vi "ZAlign_Draw_Locals_DecoFrame.vi"(8 "error in (no error)":errorcluster, 9 "Left":u32, 10 "ControlsAvailable":bool caption="Boolean", 11 "Generic in":refnum<vi>) -> (0 "error out":errorcluster, 3 "Decoration out":refnum<vi>)   [LabVIEW 2014, in "ZAlign.lvlib"]
doc: "ZAlign.lvlib:ZAlign_Draw_Locals_DecoFrame.vi\n----------------------------------------------\nDraw Locals Decoframe\n\nInputs:\n---------------------\n- error in (no error) : Cluster; \n- Left : U32; \n- Boolean : Boolean; \n- Generic in : Refnum; \n\nOutputs:\n---------------------\n- error out : Cluster; \n- Decoration out : Refnum; \n\n----------------------------------------------\n16/03/2015\nZühlke Engineering AG\nCH-8952 Schlieren\nwww.zuehlke.com"
uses:
  ZAlign.lvlib
panel:
  # "Connector Pane"
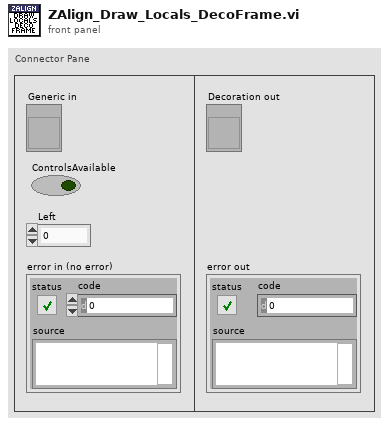
[diagram p1: front panel]
types:
  T1 = cluster{"left":i16, "top":i16, "right":i16, "bottom":i16}
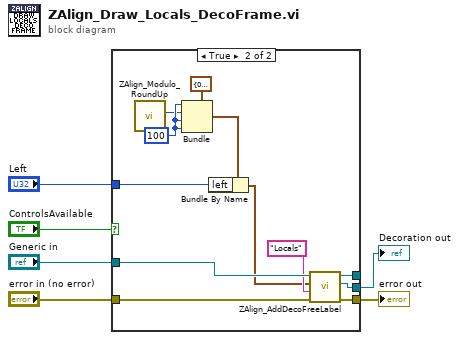
[diagram p0: block diagram]
diagram:
  n1 = case shown="True" "ControlsAvailable" {
    tunnel: "Generic in" -> [w7 w19]
    tunnel: [w7 w18] -> _
    tunnel: "Left" -> [_ w15]
    tunnel: [_ w14] -> w2
    tunnel: [_ w13] -> w3
    tunnel: "error in (no error)" -> [_ w12]
    frame False {
    }
    frame True {
      w9 = i16 100 ("y")
      n2 = call "ZAlign_Modulo_RoundUp.vi"() -> ("Grid_Size"=w8:i32)  [unwired: 10 in, 1 out]
      n3 = Bundle(cluster=T1 {"left"=0, "top"=0, "right"=0, "bottom"=0} ("rect"), "left"=w9, "top"=w8, "right"=w9, "bottom"=w9) -> (w10:T1)
      n4 = Bundle By Name(cluster=w10, "left"=w15) -> (w16:T1)
      n5 = call "ZAlign_AddDecoFreeLabel.vi"("error in (no error)"=w12, "Text"="Locals", "rect"=w16, "owner refnum"=w19) -> ("error out"=w13:errorcluster, "Decoration refnum"=w14:refnum<vi>, "owner refnumout"=w18:refnum<vi>)  [unwired: 5 in]
    }
  }
  "error out" <- w3
  "Decoration out" <- w2
